vi "Heat2D_Solve Equations.vi"(7 "LU Factor":T1, 8 "RHS":dbl[][](array[numeric]), 9 "SuperDiagonal":dbl[](array[numeric]), 10 "MainDiagonal":dbl[](array[numeric]), 11 "SubDiagonal":dbl[](array[numeric])) -> (3 "Solution Vector":dbl[][](array[numeric]))   [LabVIEW 2020, in "NI_PDE.lvlib"]
uses:
  <vilib>/gmath/NI_PDE.lvlib
  <vilib>/Analysis/7linalg.llb/Solve Linear Equations (multiple right hand).vi
  <vilib>/Analysis/NI_AALPro.lvlib
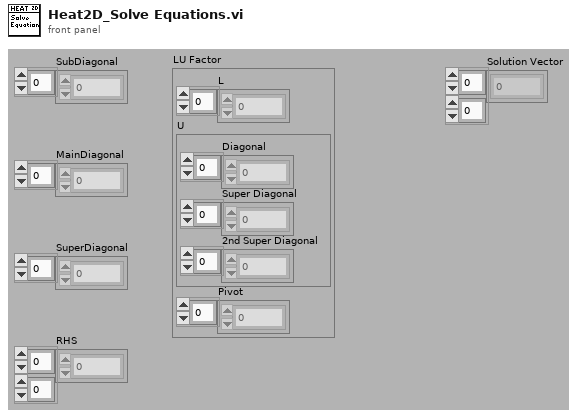
[diagram p1: front panel]
types:
  T1 = cluster{"L":dbl[], "U":cluster{"Diagonal":dbl[], "Super Diagonal":dbl[], "2nd Super Diagonal":dbl[]}, "Pivot":i32[]}
  T2 = cluster{"Diagonal":dbl[], "Super Diagonal":dbl[], "2nd Super Diagonal":dbl[]}
  T3 = typedef "NI_Matrix.lvlib/RealMatrix.ctl" = dbl[][]
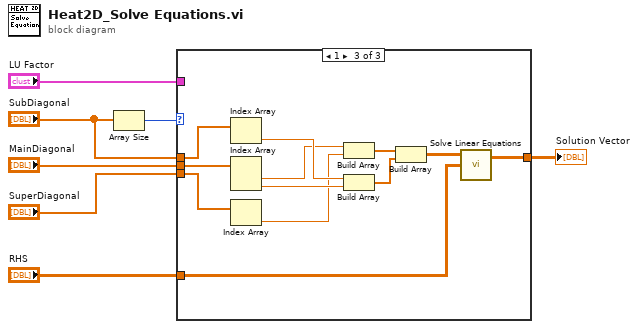
[diagram p0: block diagram]
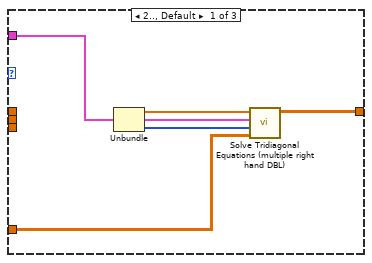
[diagram p2: hidden frame]
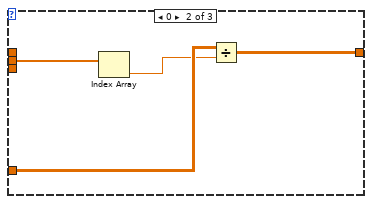
[diagram p3: hidden frame]
diagram:
  n1 = Array Size(array="SubDiagonal") -> (size(s)=w2:i32)
  n2 = case shown="1" w2 {
    tunnel: "SuperDiagonal" -> [_ _ w27]
    tunnel: "MainDiagonal" -> [_ w17 w28]
    tunnel: [w13 w14 w20] -> w5
    tunnel: "RHS" -> [w12 w16 w21]
    tunnel: "SubDiagonal" -> [_ _ w29]
    tunnel: "LU Factor" -> [w11 _ _]
    frame 2.., Default {
      n3 = Unbundle(w11) -> ("L"=w10:dbl[], "U"=w9:T2, "Pivot"=w8:i32[])
      n4 = call <vilib>:"Solve Tridiagonal Equations (multiple right hand DBL).vi"("Known Matrix"=w12, "Pivot"=w8, "U"=w9, "L"=w10) -> ("Solution Matrix"=w13:T3)  [unwired: 7 out]
    }
    frame 0 {
      n5 = Index Array(array=w17) -> (element=w15:dbl)  [unwired: 1 in]
      n6 = Divide(x=w16, y=w15) -> (x/y=w14:dbl[][])
    }
    frame 1 {
      n7 = Index Array(array=w29) -> (element=w26:dbl)  [unwired: 1 in]
      n8 = Index Array(array=w28) -> (element #1=w24:dbl, element #2=w25:dbl)  [unwired: 2 in]
      n9 = Index Array(array=w27) -> (element=w23:dbl)  [unwired: 1 in]
      n10 = Build Array(w24, w23) -> (w19:dbl[])
      n11 = Build Array(w26, w25) -> (w18:dbl[])
      n12 = Build Array(w19, w18) -> (w22:dbl[][])
      n13 = call-poly <vilib>:"Solve Linear Equations.vi"("Known Matrix"=w21, "Input Matrix"=w22) -> ("Solution Matrix"=w20:T3)  [unwired: 1 in, 1 out]
    }
  }
  "Solution Vector" <- w5
